vi "Change Tag Input B.vi"(6 "Variant":variant, 8 "error in (no error)":errorcluster, 9 "old values":string[][](array[string]), 10 "object ref in":T1, 11 "Cluster":T2) -> (0 "error out":errorcluster)   [LabVIEW 2013]
doc: "Copyright 2016 National Instruments Corporation\n\nLicensed under the Apache License, Version 2.0 (the \"License\"); you may not use this file except in compliance with the License. You may obtain a copy of the License at http://www.apache.org/licenses/LICENSE-2.0\nUnless required by applicable law or agreed to in writing, software distributed under the License is distributed on an \"AS IS\" BASIS, WITHOUT WARRANTIES OR CONDITIONS OF ANY KIND, either express or implied. See the License for the specific language governing permissions and limitations under the License."
uses:
  module/configuration/current tag file io module configuration.lvclass
  <vilib>/NI/DCAF/Tag Editor Core/Configuration Editor/Classes/Engine Parent/Engine Parent Editor Node.lvclass
  <vilib>/NI/DCAF/Tag Editor Core/Configuration Editor/Classes/Module editor node/module editor node.lvclass
  <vilib>/NI/Tag Bus Module Framework/channel/TBM channel.lvclass
  <vilib>/NI/Tag Bus/tag/tag descriptor.lvclass
  <vilib>/NI/DCAF Table API/Table Manager/Cell Change.ctl
  <vilib>/NI/DCAF Table API/Table Manager.lvlib
  <vilib>/NI/DCAF Table API/Table Manager/object ref.ctl
  <vilib>/NI/DCAF Table API/Table Manager/Table Manager.lvclass
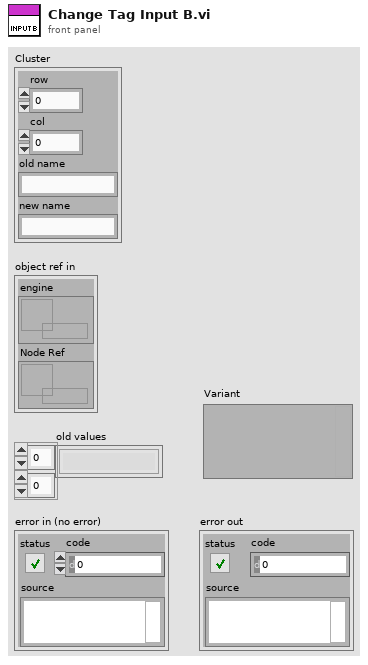
[diagram p1: front panel]
types:
  T1 = typedef "Table Manager.lvlib/Table Manager.lvclass/object ref.ctl" = cluster{"engine":refnum<data-value>, "Node Ref":refnum<data-value>}
  T2 = typedef "Table Manager.lvlib/Cell Change.ctl" = cluster{"row":i32, "col":i32, "old name":string, "new name":string}
  T3 = typedef "current tag file io module configuration.lvclass/tag configuration.ctl" = cluster{"name":string, "data type":T4, "channel":refnum<class "TBM channel.lvclass">}
  T4 = typedef "tag bus.lvlib/tag descriptor.lvclass/Data Type.ctl" = enum16{"Double", "Single", "I64", "I32", "I16", "I8", "U64", "U32", "U16", "U8", "Boolean", "String", "Array of Double", "Array of Single", "Array of I64", "Array of I32", "Array of I16", "Array of I8", "Array of U64", "Array of U32", "Array of U16", "Array of U8", "Array of Boolean", "Array of String"}
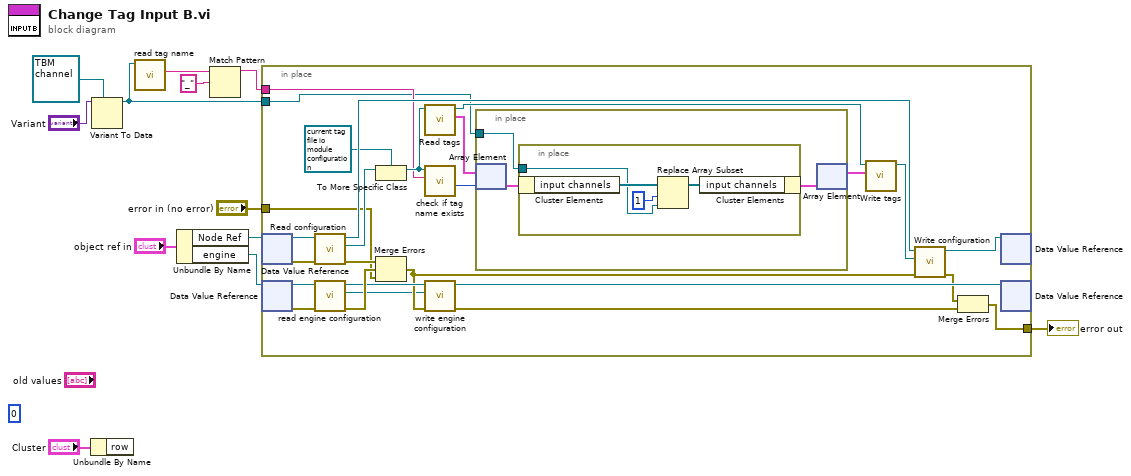
[diagram p0: block diagram]
diagram:
  (unwired) 0 ("disabled index (col)")
  n1 = Unbundle By Name("Cluster") -> ()  [unwired: 1 out]
  n2 = Variant To Data(type=refnum<class "TBM channel.lvclass"> refnum ("output"), Variant="Variant") -> (data=w2:refnum<class "TBM channel.lvclass">)  [unwired: 1 in, 1 out]
  n3 = call <vilib>:"read tag name.vi"("system tag in"=w2) -> ("name"=w4:string)  [unwired: 8 in, 2 out]
  n4 = Unbundle By Name("object ref in") -> ("Node Ref"=w8:refnum<data-value>, "engine"=w7:refnum<data-value>)
  n5 = Match Pattern(string=w4, regular expression="_") -> (before substring=w1:string)  [unwired: 1 in, 3 out]
  n6 = in-place {
    in-place-border: [w30] -> w12
    in-place-border: "error in (no error)" -> [w22]
    in-place-border: w1 -> [w16]
    in-place-border: w2 -> [w13]
    n7 = in-place-dvr #1(w8) -> (w27:refnum<class "module editor node.lvclass">, w29:errorcluster)
    n8 = in-place-dvr #2(w7) -> (w37:refnum<class "Engine Parent Editor Node.lvclass">, w38:errorcluster)
    n9 = call-dynamic "Read configuration.vi"("error in"=w29, "NISE_CEF_serializable node in"=w27) -> ("error out"=w28:errorcluster, "configuration"=w25:refnum<class "NISE_CEF_serializable configuration.lvclass">, "NISE_CEF_serializable node out"=w26:refnum<class "module editor node.lvclass">)  [unwired: 7 in]
    n10 = call <vilib>:"read engine configuration.vi"("error in"=w38, "Engine Parent Editor Node in"=w37) -> ("error out"=w34:errorcluster, "engine configuration"=w14:refnum<class "engine configuration.lvclass">, "Engine Parent Editor Node out"=w33:refnum<class "Engine Parent Editor Node.lvclass">)  [unwired: 7 in]
    n11 = To More Specific Class(target class=refnum<class "current tag file io module configuration.lvclass"> refnum ("tag select module configuration"), reference=w25) -> (specific class reference=w21:refnum<class "current tag file io module configuration.lvclass">)  [unwired: 1 in, 1 out]
    n12 = Merge Errors(w28, w34, w22) -> (w24:errorcluster)
    n13 = call "Read tags.vi"("current tag file io module configuration in"=w21) -> ("tags"=w20:T3[], "current tag file io module configuration out"=w18:refnum<class "current tag file io module configuration.lvclass">)  [unwired: 8 in, 1 out]
    n14 = call "check if tag name exists.vi"("name to locate"=w16, "current tag file io module configuration in"=w21) -> ("index"=w17:i32)  [unwired: 6 in, 3 out]
    n15 = call <vilib>:"write engine configuration.vi"("error in"=w24, "engine configuration"=w14, "Engine Parent Editor Node in"=w33) -> ("error out"=w32:errorcluster, "Engine Parent Editor Node out"=w36:refnum<class "Engine Parent Editor Node.lvclass">)  [unwired: 7 in]
    n16 = in-place {
      in-place-border: w13 -> [w39]
      n17 = in-place-array #3(w20, w17) -> (w41:T3)
      n18 = in-place {
        in-place-border: w39 -> [w42]
        n19 = in-place-cluster #4(w41) -> ("input channels"=w45:refnum<class "TBM channel.lvclass">[])
        n20 = Replace Array Subset(array=w45, new element=w42, index=1) -> (w44:refnum<class "TBM channel.lvclass">[])
        n21 = in-place-cluster #4("input channels"=w44) -> (w40:T3)
      }
      n22 = in-place-array #3(w40) -> (w19:T3[])  [unwired: 1 out]
    }
    n23 = call "Write tags.vi"("tags"=w19, "current tag file io module configuration in"=w18) -> ("current tag file io module configuration out"=w15:refnum<class "current tag file io module configuration.lvclass">)  [unwired: 8 in, 1 out]
    n24 = call-dynamic "Write configuration.vi"("error in"=w24, "configuration"=w15, "NISE_CEF_serializable node in"=w26) -> ("error out"=w31:errorcluster, "NISE_CEF_serializable node out"=w35:refnum<class "module editor node.lvclass">)  [unwired: 7 in]
    n25 = Merge Errors(w31, w32) -> (w30:errorcluster)
    n26 = in-place-dvr #1(w35) -> ()  [unwired: 2 out]
    n27 = in-place-dvr #2(w36) -> ()  [unwired: 2 out]
  }
  "error out" <- w12
